vi "check_last_time_current_pos.vi"(8 "error in (no error)":errorcluster caption="错误输入（无错误）", 11 "MotorSystem 输入":refnum<class "MotorSystem.lvclass">) -> (0 "error out":errorcluster caption="错误输出", 3 "MotorSystem 输出":refnum<class "MotorSystem.lvclass">)   [LabVIEW 2016, in "MotionControl_UFO_3DOF.lvlib" / "MotorSystem.lvclass"]
uses:
  <userlib>/MotionControl_UFO_3DOF/MotorSystem/MotorSystem.lvclass
  <userlib>/MotionControl_UFO_3DOF/MotorSystem/MotorSystem.lvclass/MotorSystem.ctl
  <vilib>/Utility/config.llb/Read Key (I32).vi
  <userlib>/MotionControl_UFO_3DOF/OneMotion/OneMotion.lvclass
  <vilib>/Utility/config.llb/NI_LVConfig.lvlib
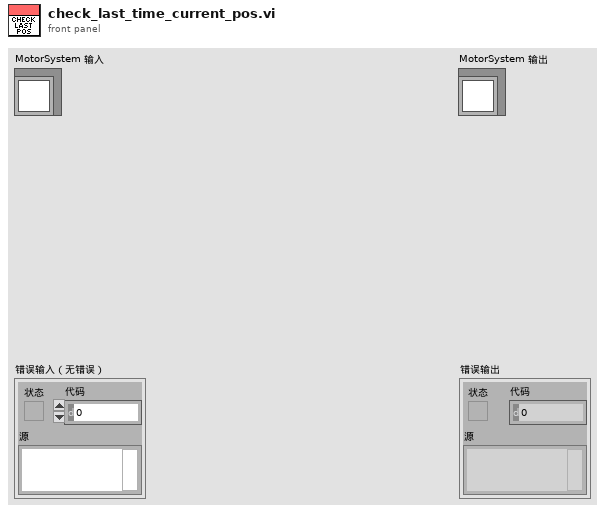
[diagram p1: front panel]
types:
  T1 = typedef "NI_LVConfig.lvlib/Config Data RefNum.ctl" = refnum<k1>
  T2 = typedef "MotionControl_UFO_3DOF.lvlib/MotorSystem.lvclass/MotionCluster.ctl" = cluster{"OneMotion.lvclass":refnum<class "OneMotion.lvclass">, "connected?":bool, "default enabled?":bool, "enabled?":bool}
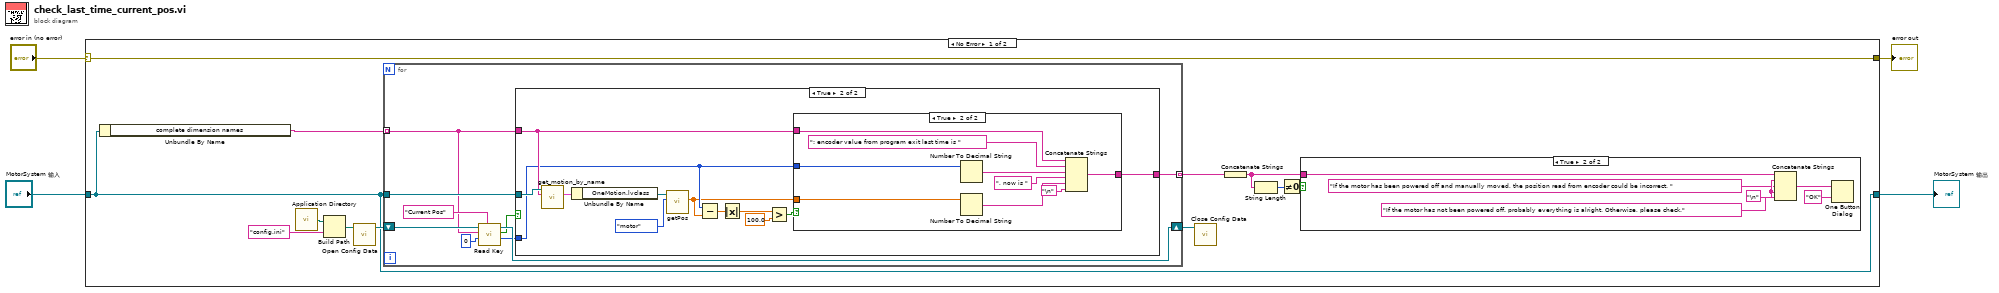
[diagram p0: block diagram]
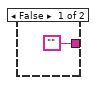
[diagram p3: hidden frame]
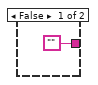
[diagram p4: hidden frame]
diagram:
  n1 = case shown="No Error" "error in (no error)" {
    selector: "error in (no error)" -> [w16 w56]
    tunnel: [w16 w56] -> w3
    tunnel: [w6 w55] -> w1
    tunnel: "MotorSystem 输入" -> [w6 w55]
    frame No Error {
      n2 = Unbundle By Name(w6) -> ("complete dimension names"=w5:string[])
      n3 = call <vilib>:"Application Directory.vi"() -> ("Application Directory"=w7:path)
      n4 = Build Path(base path=w7, name or relative path="config.ini" ("名称或相对路径")) -> (appended path=w9:path)
      n5 = call <vilib>:"Open Config Data.vi"("configuration file path"=w9) -> ("refnum"=w10:T1)  [unwired: 8 in, 2 out]
      n6 = for {
        tunnel: w5 -> [w25] mode=indexing
        shift-right: [w29] -> w11
        shift-left: w10 -> [w30]
        tunnel: w6 -> [w26]
        tunnel: [w23] -> w14 mode=indexing
        n7 = call-poly <vilib>:"Read Key.vi"("section"="Current Pos", "default value"=0, "key"=w25, "refnum"=w30) -> ("value"=w24:i32, "found?"=w27:bool, "refnum out"=w29:T1)  [unwired: 4 in, 1 out]
        n8 = case shown="True" w27 {
          tunnel: w26 -> [_ w44]
          tunnel: w25 -> [_ w36]
          tunnel: w24 -> [_ w35]
          tunnel: ["" w33] -> w23
          frame False {
          }
          frame True {
            n9 = call <userlib>:"get_motion_by_name.vi"("name"=w36, "MotorSystem in"=w44) -> ("motion cluster"=w43:T2)  [unwired: 7 in, 2 out]
            n10 = Unbundle By Name(w43) -> ("OneMotion.lvclass"=w42:refnum<class "OneMotion.lvclass">)
            n11 = call <userlib>:"getPos.vi"("lab or motor"=enum16{"lab", "motor"}."motor", "OneMotion 输入"=w42) -> ("pos"=w34:dbl)  [unwired: 7 in, 2 out]
            n12 = Subtract(x=w35, y=w34) -> (x-y=w40:dbl)
            n13 = Absolute Value(x=w40) -> (abs(x)=w39:dbl)
            n14 = Greater?(x=w39, y=100.0) -> (0:w37:bool)
            n15 = case shown="True" w37 {
              tunnel: w36 -> [_ w54]
              tunnel: w35 -> [_ w52]
              tunnel: w34 -> [_ w49]
              tunnel: ["" w46] -> w33
              frame False {
              }
              frame True {
                n16 = Number To Decimal String(number=w52) -> (decimal integer string=w51:string)  [unwired: 1 in]
                n17 = Number To Decimal String(number=w49) -> (decimal integer string=w48:string)  [unwired: 1 in]
                n18 = Concatenate Strings(w54, ": encoder value from program exit last time is ", w51, ", now is ", w48, "\n") -> (w46:string)
              }
            }
          }
        }
      }
      n19 = call <vilib>:"Close Config Data.vi"("refnum"=w11) -> ()  [unwired: 9 in, 2 out]
      n20 = Concatenate Strings(w14) -> (w15:string)
      n21 = String Length(string=w15) -> (length=w12:i32)
      n22 = Not Equal To 0?(x=w12) -> (x != 0?=w13:bool)
      n23 = case shown="True" w13 {
        tunnel: w15 -> [_ w21]
        frame False {
        }
        frame True {
          w18 = "\n"
          n24 = Concatenate Strings(w21, w18, "If the motor has been powered off and manually moved, the position read from encoder could be incorrect. ", w18, "If the motor has not been powered off. probably everything is alright. Otherwise, please check.") -> (w20:string)
          n25 = One Button Dialog(message=w20, button name ("OK")="OK" ("按钮名称（“确定”）")) -> ()  [unwired: 1 out]
        }
      }
    }
    frame Error {
    }
  }
  "error out" <- w3
  "MotorSystem 输出" <- w1
